vi "Write Text.vi"(8 "error in (no error)":errorcluster, 9 "Text":string, 11 "Character LCD in":refnum<class "Char LCD.lvclass">) -> (0 "error out":errorcluster, 3 "Character LCD out":refnum<class "Char LCD.lvclass">)   [LabVIEW 2020, in "CTI-Peripheral.lvlib" / "Char LCD.lvclass"]
uses:
  Char LCD.lvclass
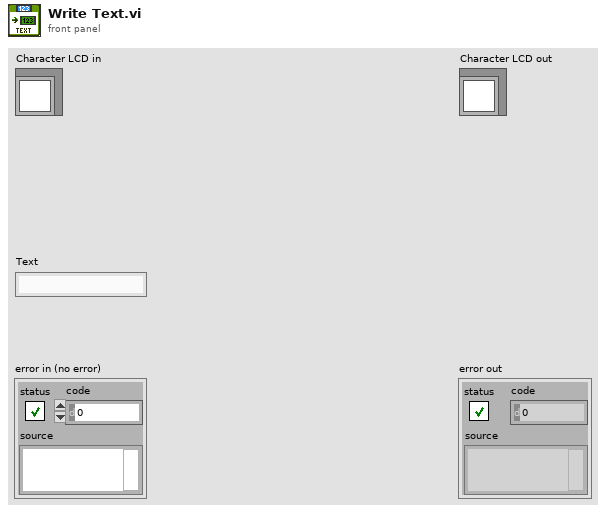
[diagram p1: front panel]
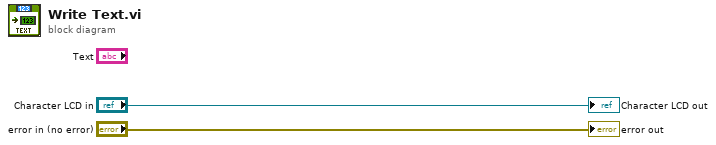
[diagram p0: block diagram]
diagram:
  "error out" <- "error in (no error)"
  "Character LCD out" <- "Character LCD in"
